vi "FPGA_target_set_output.vi"(3 "tick_count_in":u32, 4 "data_in":T1, 6 "new_data_in":T1, 7 "set_outputs":bool=TRUE, 11 "C1_data":T2) -> (17 "tick_count_out":u32, 18 "data_out":T1)   [LabVIEW 2014]
doc: "writes a 64 bit pattern to the output lines"
uses:
  FPGA_32BitPattern_data_type.ctl
  FPGA_cmd_data_type.ctl
  <vilib>/rvi/eio/common/nirviEmuTemplateMethod_errors.vi
  <vilib>/eio/EIONode/EIONode.xnode
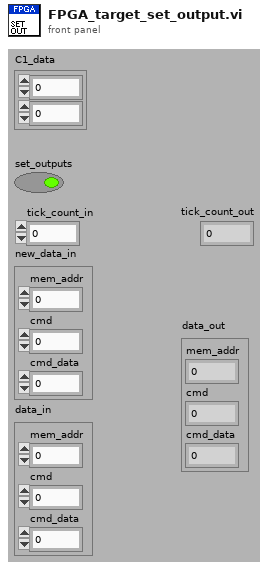
[diagram p1: front panel]
types:
  T1 = typedef "FPGA_cmd_data_type.ctl" = cluster{"mem_addr":u32, "cmd":u8, "cmd_data":u32}
  T2 = typedef "FPGA_32BitPattern_data_type.ctl" = cluster{"port0":u8, "port1":u8}
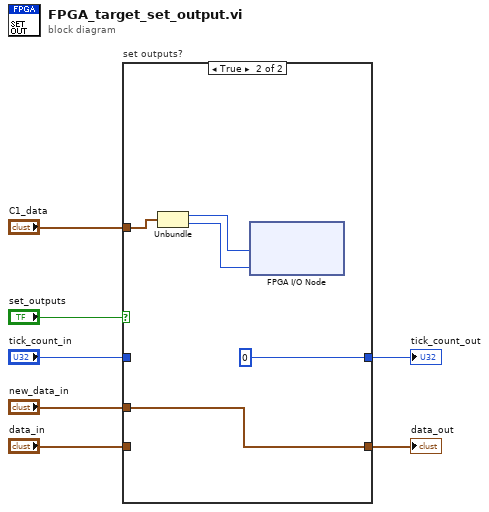
[diagram p0: block diagram]
diagram:
  n1 = case "set outputs?" shown="True" "set_outputs" {
    tunnel: [w9 u32 0] -> w7
    tunnel: "tick_count_in" -> [w9 _]
    tunnel: "C1_data" -> [_ w12]
    tunnel: "new_data_in" -> [_ w10]
    tunnel: [w8 w10] -> w2
    tunnel: "data_in" -> [w8 _]
    frame False {
    }
    frame True {
      n2 = Unbundle(w12) -> ("port0"=w13:u8, "port1"=w14:u8)
      n3 = xnode ("FPGA I/O Node")("DO_08-15"=w13, "DO_00-07"=w14) -> ()  [unwired: 2 in, 2 out]
    }
  }
  "tick_count_out" <- w7
  "data_out" <- w2
